vi "Teleop.vi"(10 "Match Info":T1={"Autonomous Elapsed Seconds"=0.0, "TeleOp Elapsed Seconds"=0.0, "Disabled Elapsed Seconds"=0.0, "Visited Autonomous"=FALSE, "Visited TeleOp"=FALSE, "Visited Disabled"=FALSE, "Autonomous Settings"={"Autonomous Style"=enum."Independent", "VI Refnum"=refnum}}, 11 "Call Context":T2) -> ()   [LabVIEW 2020]
doc: "This VI is called for each TeleOp packet received from the DS where the robot is not disabled. It is often used to read from the joysticks and update I/O or to update setpoints for timed control loops. It should complete and return within 20 milliseconds or it may miss DS packets."
uses:
  <vilib>/Rock Robotics/WPI/DriverStation/WPI_DriverStationDerivedRobotMode.ctl
  <vilib>/Rock Robotics/WPI/DriverStation/WPI_DriverStationMatch Info.ctl
  <vilib>/Rock Robotics/WPI/ThirdParty/Phoenix-LabVIEW/Motor Controller/Controls/CTRE_Phoenix_MotorControl_ControlMode.ctl
  <vilib>/Rock Robotics/WPI/Solenoid/WPI_SolenoidValue.ctl
  <vilib>/Rock Robotics/WPI/Utilities/WPI_GetSetVariantRefNum.vi
  <vilib>/Rock Robotics/Network Tables/NT Write Boolean Array.vi
  <vilib>/Rock Robotics/Network Tables/NT Write Numeric Array.vi
  <vilib>/Rock Robotics/Network Tables/NT Read Boolean.vi
  <vilib>/Rock Robotics/WPI/Solenoid/WPI_SolenoidSetEnum.vi
  <vilib>/Rock Robotics/WPI/ThirdParty/Phoenix-LabVIEW/Motor Controller/Get/CTRE_Phoenix_MotorController_IntegratedSensorData_TalonFX.vi
  <vilib>/Rock Robotics/WPI/ThirdParty/Phoenix-LabVIEW/Motor Controller/Get/CTRE_Phoenix_MotorController_GetLimitSwitchStates.vi
  <vilib>/Rock Robotics/WPI/ThirdParty/Phoenix-LabVIEW/Motor Controller/Sensor/CTRE_Phoenix_MotorControl_SetIntegratedSensorPosition_TalonFX.vi
  <vilib>/Rock Robotics/Network Tables/NT Write Number.vi
  Lime.vi
  <vilib>/Rock Robotics/WPI/RobotDrive/WPI_RobotDriveMecanumDrive_Cartesian.vi
panel:
  in  "Numeric":dbl=-0.7 format="%#_13g"
  in  "Auger Speed":dbl=-0.8
  out "Present Text":string
  in  "Total Time":dbl=0.9 format="%#_13g"
  in  "Time Low":dbl=0.6 format="%#_13g"
  in  "Slowmode Speed":dbl=0.33
  out "Compressor Running":bool
  out "Enabled":bool
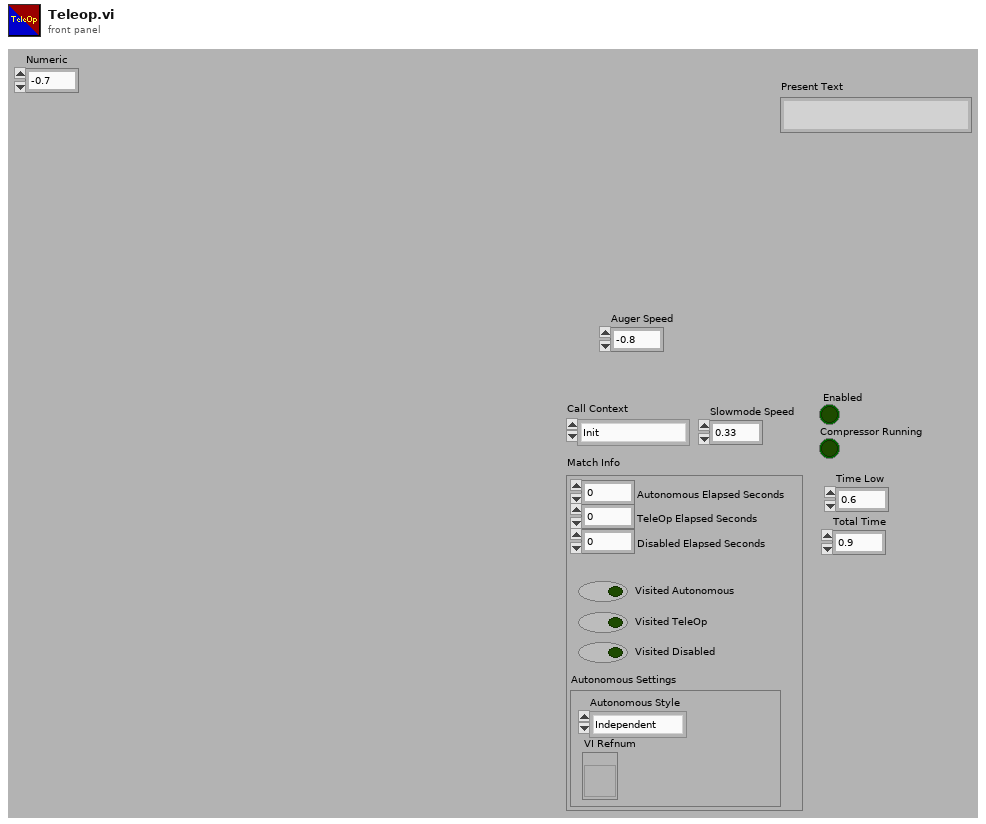
[diagram p1: front panel]
types:
  T1 = typedef "WPI_DriverStationMatch Info.ctl" = cluster{"Autonomous Elapsed Seconds":dbl, "TeleOp Elapsed Seconds":dbl, "Disabled Elapsed Seconds":dbl, "Visited Autonomous":bool, "Visited TeleOp":bool, "Visited Disabled":bool, "Autonomous Settings":cluster{"Autonomous Style":enum16{"Iterative", "Independent"}, "VI Refnum":refnum<vi>}}
  T2 = typedef "WPI_DriverStationDerivedRobotMode.ctl" = enum16{"Init", "Execute", "Stop"}
  T3 = typedef "WPI_SolenoidValue.ctl" = enum16{"Off", "On", "Forward", "Reverse"}
  T4 = typedef "CTRE_Phoenix_MotorControl_ControlMode.ctl" = u16
  T5 = typedef "WPI_JoystickDevRef.ctl" = cluster{"Device":T6}
  T6 = typedef "WPI_JoystickDeviceEnum.ctl" = enum16{"USB 0", "USB 1", "USB 2", "USB 3", "USB 4", "USB 5"}
  T7 = typedef "WPI_CompressorDevRef.ctl" = cluster{"DevStatus":errorcluster, "Pneumatics Control Module":u8}
  T8 = typedef "WPI_RobotDriveDevRef.ctl" = cluster{"DevStatus":errorcluster, "Motors[]":T9[], "Square Inputs":bool, "Max Output":dbl}
  T9 = typedef "WPI_MotorControlDeviceRef.ctl" = cluster{"DeviceStatus":errorcluster, "Type":T10, "PWM":cluster{"PWM Channel":T11, "DeadBand":T12}, "CAN":cluster{"Device Number":u8, "SetOutput VI Ref":variant, "GetOutput VI Ref":variant, "Enable VI Ref":variant, "Disable VI Ref":variant, "Data":variant}, "Invert":bool, "DIO PWM":cluster{"PWM \"Enable\" Channel":T11, "DIOChannel":T13, "PWM Rate":dbl}}
  T10 = typedef "WPI_MotorControlType.ctl" = enum16{"PWM", "CAN", "DIO PWM"}
  T11 = typedef "FPGA_DIOPWMChannel.ctl" = enum8{"PWM 0", "PWM 1", "PWM 2", "PWM 3", "PWM 4", "PWM 5", "PWM 6", "PWM 7", "PWM 8", "PWM 9", "PWM MXP 0", "PWM MXP 1", "PWM MXP 2", "PWM MXP 3", "PWM MXP 4", "PWM MXP 5", "PWM MXP 6", "PWM MXP 7", "PWM MXP 8", "PWM MXP 9", "Invalid"}
  T12 = typedef "WPI_PWMDeadband.ctl" = cluster{"Name":string, "maxPositivePwm":i32, "minPositivePwm":i32, "centerPwm":i32, "maxNegativePwm":i32, "minNegativePwm":i32, "angularRange":u16}
  T13 = typedef "FPGA_DIOChannel.ctl" = enum8{"DIO 0", "DIO 1", "DIO 2", "DIO 3", "DIO 4", "DIO 5", "DIO 6", "DIO 7", "DIO 8", "DIO 9", "DIO MXP 0", "DIO MXP 1", "DIO MXP 2", "DIO MXP 3", "DIO MXP 4", "DIO MXP 5", "DIO MXP 6", "DIO MXP 7", "DIO MXP 8", "DIO MXP 9", "DIO MXP 10", "DIO MXP 11", "DIO MXP 12", "DIO MXP 13", "DIO MXP 14", "DIO MXP 15", "SPI Port CS1", "SPI Port CS2", "SPI Port CS3", "SPI Port MISO", "SPI Port MOSI", "Invalid"}
  T14 = typedef "WPI_DigitalInputDevRef.ctl" = cluster{"DevStatus":errorcluster, "DIO Channel":T13}
  T15 = typedef "WPI_SolenoidDevRef.ctl" = cluster{"DevStatus":errorcluster, "Pneumatics Control Module":u8, "Forward Solenoid Channel":T16, "Reverse Solenoid Channel":T16}
  T16 = typedef "WPI_SolenoidChannel.ctl" = enum8{"Solenoid 0", "Solenoid 1", "Solenoid 2", "Solenoid 3", "Solenoid 4", "Solenoid 5", "Solenoid 6", "Solenoid 7", "Solenoid 8", "Solenoid 9", "Solenoid 10", "Solenoid 11", "Solenoid 12", "Solenoid 13", "Solenoid 14", "Solenoid 15", "Invalid"}
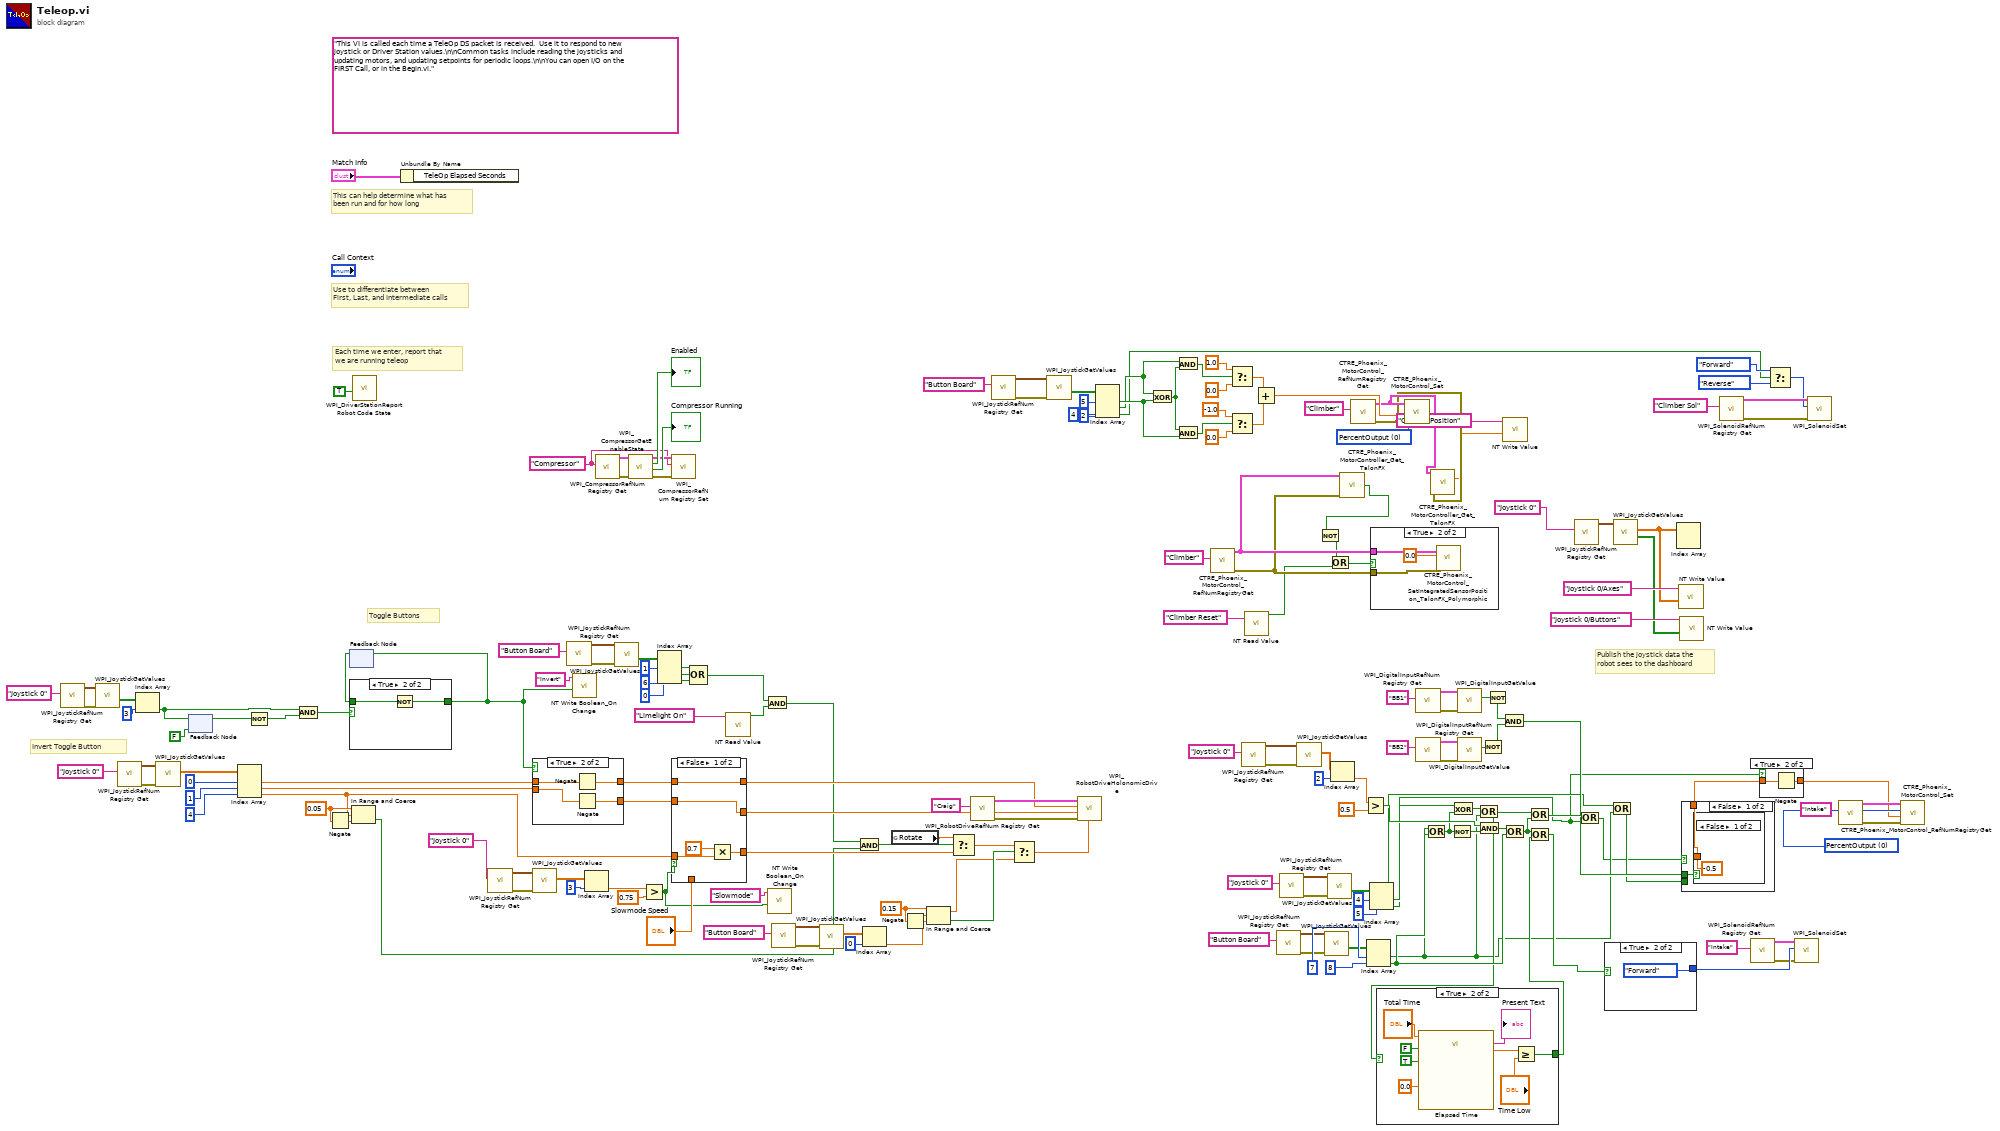
[diagram p0: block diagram]
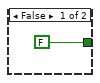
[diagram p4: hidden frame]
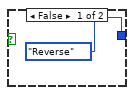
[diagram p5: hidden frame]
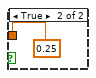
[diagram p6: hidden frame]
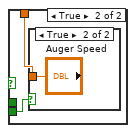
[diagram p7: hidden frame]
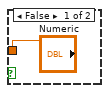
[diagram p8: hidden frame]
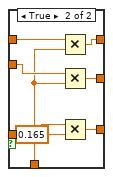
[diagram p9: hidden frame]
diagram:
  w41 = T4 0 items=["PercentOutput"=0, "Position"=1, "Velocity"=2, "Current"=3, "Follower"=5, "MotionProfile"=6, "MotionMagic"=7, "MotionProfileArc"=10, "Disabled"=15] ("Control Mode")
  w45 = 0.15 ("upper limit")
  w56 = 0.05 ("upper limit")
  w91 = T4 0 items=["PercentOutput"=0, "Position"=1, "Velocity"=2, "Current"=3, "Follower"=5, "MotionProfile"=6, "MotionMagic"=7, "MotionProfileArc"=10, "Disabled"=15] ("Control Mode")
  w169 = "Compressor" ("refnum name")
  (unwired) "This VI is called each time a TeleOp DS packet is received.  Use it to respond to new joystick or Driver Station values.\n\nCommon tasks include reading the joysticks and updating motors, and updating setpoints for periodic loops.\n\nYou can open I/O on the FIRST Call, or in the Begin.vi."
  # "Invert Toggle Button"
  # "Toggle Buttons"
  # "Publish the joystick data the\nrobot sees to the dashboard"
  # "Each time we enter, report that\nwe are running teleop"
  # "Use to differentiate between\nFirst, Last, and Intermediate calls"
  # "This can help determine what has\nbeen run and for how long"
  n1 = call <vilib>:"WPI_JoystickRefNum Registry Get.vi"("refnum name"="Joystick 0") -> ("error out"=w158:errorcluster, "JoystickDevRef"=w147:T5)  [unwired: 9 in]
  n2 = call <vilib>:"WPI_JoystickGetValues.vi"("error in (no error)"=w158, "JoystickDevRef"=w147) -> ("Buttons"=w155:bool[])  [unwired: 5 in, 4 out]
  n3 = call <vilib>:"WPI_JoystickRefNum Registry Get.vi"("refnum name"="Joystick 0") -> ("error out"=w165:errorcluster, "JoystickDevRef"=w166:T5)  [unwired: 9 in]
  n4 = Index Array(array=w155, index=3) -> (element=w149:bool)
  n5 = call <vilib>:"WPI_JoystickGetValues.vi"("error in (no error)"=w165, "JoystickDevRef"=w166) -> ("Axes"=w162:dbl[])  [unwired: 5 in, 4 out]
  n6 = feedback #1(FALSE) -> (w151:bool)
  n7 = feedback-in #1(w149) -> ()
  n8 = Index Array(array=w162, index #1=0 ("index"), index #2=1 ("index"), index #3=4 ("index")) -> (element #1=w148:dbl, element #2=w135:dbl, element #3=w53:dbl)
  n9 = Not(x=w151) -> (.not. x?=w152:bool)
  n10 = And(x=w149, y=w152) -> (x .and. y?=w153:bool)
  n11 = Negate(x=w56) -> (-x=w57:dbl)
  n12 = feedback #2() -> (w154:bool)  [unwired: 1 in]
  n13 = case shown="True" w153 {
    tunnel: w154 -> [w184 w186]
    tunnel: [w184 w185] -> w134
    frame False {
    }
    frame True {
      n14 = Not(x=w186) -> (.not. x?=w185:bool)
    }
  }
  n15 = feedback-in #2(w134) -> ()
  n16 = In Range and Coerce(upper limit=w56, x=w53, lower limit=w57) -> (In Range?=w54:bool)  [unwired: 1 out]
  n17 = call <vilib>:"WPI_DriverStationReport Robot Code State.vi"("TeleOp"=TRUE ("Autonomous")) -> ()  [unwired: 10 in, 1 out]
  n18 = Unbundle By Name("Match Info") -> ()  [unwired: 1 out]
  n19 = call <vilib>:"WPI_JoystickRefNum Registry Get.vi"("refnum name"="Joystick 0") -> ("error out"=w141:errorcluster, "JoystickDevRef"=w144:T5)  [unwired: 9 in]
  n20 = case shown="True" w134 {
    tunnel: [w188 w189] -> w146
    tunnel: w148 -> [w188 w190]
    tunnel: [w187 w191] -> w145
    tunnel: w135 -> [w187 w192]
    frame False {
    }
    frame True {
      n21 = Negate(x=w190) -> (-x=w189:dbl)
      n22 = Negate(x=w192) -> (-x=w191:dbl)
    }
  }
  n23 = call <vilib>:"WPI_JoystickGetValues.vi"("error in (no error)"=w141, "JoystickDevRef"=w144) -> ("Axes"=w140:dbl[])  [unwired: 5 in, 4 out]
  n24 = call <vilib>:"WPI_JoystickRefNum Registry Get.vi"("refnum name"="Button Board") -> ("error out"=w129:errorcluster, "JoystickDevRef"=w127:T5)  [unwired: 9 in]
  n25 = call "NT Write Boolean_On Change.vi"("Boolean"=w134, "Name"="Invert") -> ()  [unwired: 9 in, 1 out]
  n26 = Index Array(array=w140, index=3) -> (element=w139:dbl)
  n27 = call <vilib>:"WPI_CompressorRefNum Registry Get.vi"("refnum name"=w169) -> ("error out"=w173:errorcluster, "CompressorDevRef"=w172:T7)  [unwired: 9 in]
  n28 = call <vilib>:"WPI_JoystickGetValues.vi"("error in (no error)"=w129, "JoystickDevRef"=w127) -> ("Buttons"=w128:bool[])  [unwired: 5 in, 4 out]
  n29 = call <vilib>:"WPI_CompressorGetEnableState.vi"("error in (no error)"=w173, "CompressorDevRef"=w172) -> ("error out"=w170:errorcluster, "Compressor Running"=→"Compressor Running":bool, "Enabled"=→"Enabled":bool, "CompressorDevRef"=w171:T7)  [unwired: 3 in, 3 out]
  n30 = Greater?(x=w139, y=0.75) -> (0:w131:bool)
  n31 = Index Array(array=w128, index #1=1 ("index"), index #2=6 ("index"), index #3=0 ("index")) -> (element #1=w120:bool, element #2=w122:bool, element #3=w121:bool)
  n32 = call <vilib>:"WPI_CompressorRefNum Registry Set.vi"("error in (no error)"=w170, "refnum name"=w169, "CompressorDevRef"=w171) -> ()  [unwired: 7 in, 2 out]
  n33 = case shown="False" w131 {
    tunnel: w53 -> [w197 w205]
    tunnel: [w194 w204] -> w59
    tunnel: w146 -> [w196 w203]
    tunnel: [w196 w202] -> w137
    tunnel: w145 -> [w195 w201]
    tunnel: [w195 w200] -> w123
    tunnel: "Slowmode Speed" -> [_ w199]
    frame False {
      n34 = Multiply(x=0.7, y=w197) -> (x*y=w194:dbl)
    }
    frame True {
      n35 = Multiply(x=w203, y=w199) -> (x*y=w202:dbl)
      n36 = Multiply(x=w201, y=w199) -> (x*y=w200:dbl)
      n37 = Multiply(x=w205, y=0.165) -> (x*y=w204:dbl)
    }
  }
  n38 = Compound Arithmetic op=OR(w120, w122, w121) -> (w117:bool)
  n39 = call-poly <vilib>:"NT Read Value.vi"("Name"="Limelight On") -> ("Boolean"=w119:bool)  [unwired: 9 in, 1 out]
  n40 = And(x=w117, y=w119) -> (x .and. y?=w61:bool)
  n41 = call "NT Write Boolean_On Change.vi"("Boolean"=w131, "Name"="Slowmode") -> ()  [unwired: 9 in, 1 out]
  n42 = call <vilib>:"WPI_JoystickRefNum Registry Get.vi"("refnum name"="Button Board") -> ("error out"=w50:errorcluster, "JoystickDevRef"=w51:T5)  [unwired: 9 in]
  n43 = call <vilib>:"WPI_JoystickGetValues.vi"("error in (no error)"=w50, "JoystickDevRef"=w51) -> ("Axes"=w48:dbl[])  [unwired: 5 in, 4 out]
  n44 = And(x=w61, y=w54) -> (x .and. y?=w55:bool)
  n45 = Index Array(array=w48, index=0) -> (element=w44:dbl)
  n46 = global read "Lime.vi" "Rotate"() -> (w60:dbl)
  n47 = Negate(x=w45) -> (-x=w47:dbl)
  n48 = In Range and Coerce(upper limit=w45, x=w44, lower limit=w47) -> (coerced(x)=w42:dbl, In Range?=w46:bool)
  n49 = Select(t=w60, s=w55, f=w59) -> (s? t:f=w58:dbl)
  n50 = call <vilib>:"WPI_RobotDriveRefNum Registry Get.vi"("refnum name"="Craig") -> ("error out"=w167:errorcluster, "RobotDriveDevRef"=w168:T8)  [unwired: 9 in]
  n51 = call <vilib>:"WPI_JoystickRefNum Registry Get.vi"("refnum name"="Button Board") -> ("error out"=w38:errorcluster, "JoystickDevRef"=w39:T5)  [unwired: 9 in]
  n52 = Select(t=w58, s=w46, f=w42) -> (s? t:f=w43:dbl)
  n53 = call <vilib>:"WPI_JoystickGetValues.vi"("error in (no error)"=w38, "JoystickDevRef"=w39) -> ("Buttons"=w36:bool[])  [unwired: 5 in, 4 out]
  n54 = call-poly <vilib>:"WPI_RobotDriveHolonomicDrive.vi"("Rotation"=w43, "error in (no error)"=w167, "Y"=w123, "X"=w137, "RobotDriveDevRef"=w168) -> ()  [unwired: 4 in, 3 out]
  n55 = Index Array(array=w36, index #1=5 ("index"), index #2=2 ("index"), index #3=4 ("index")) -> (element #1=w24:bool, element #2=w23:bool, element #3=w2:bool)
  n56 = Exclusive Or(1:w24, 2:w23) -> (0:w27:bool)
  n57 = And(x=w23, y=w27) -> (x .and. y?=w29:bool)
  n58 = And(x=w27, y=w24) -> (x .and. y?=w28:bool)
  n59 = call <vilib>:"CTRE_Phoenix_MotorControl_RefNumRegistryGet.vi"("refnum name"="Climber") -> ("error out"=w19:errorcluster, "PhoenixMotorControlDevRef"=w20:T9)  [unwired: 9 in]
  n60 = Select(t=1.0, s=w29, f=0.0) -> (s? t:f=w25:dbl)
  n61 = Select(t=-1.0, s=w28, f=0.0) -> (s? t:f=w26:dbl)
  n62 = call <vilib>:"WPI_JoystickRefNum Registry Get.vi"("refnum name"="Joystick 0") -> ("error out"=w96:errorcluster, "JoystickDevRef"=w95:T5)  [unwired: 9 in]
  n63 = call-poly <vilib>:"NT Read Value.vi"("Name"="Climber Reset") -> ("Boolean"=w15:bool)  [unwired: 9 in, 1 out]
  n64 = Add(x=w25, y=w26) -> (x+y=w22:dbl)
  n65 = call <vilib>:"WPI_JoystickRefNum Registry Get.vi"("refnum name"="Button Board") -> ("error out"=w79:errorcluster, "JoystickDevRef"=w77:T5)  [unwired: 9 in]
  n66 = call <vilib>:"WPI_JoystickRefNum Registry Get.vi"("refnum name"="Joystick 0") -> ("error out"=w102:errorcluster, "JoystickDevRef"=w104:T5)  [unwired: 9 in]
  n67 = call <vilib>:"WPI_JoystickGetValues.vi"("error in (no error)"=w96, "JoystickDevRef"=w95) -> ("Axes"=w97:dbl[])  [unwired: 5 in, 4 out]
  n68 = call <vilib>:"WPI_JoystickGetValues.vi"("error in (no error)"=w79, "JoystickDevRef"=w77) -> ("Buttons"=w78:bool[])  [unwired: 5 in, 4 out]
  n69 = call <vilib>:"WPI_JoystickGetValues.vi"("error in (no error)"=w102, "JoystickDevRef"=w104) -> ("Buttons"=w103:bool[])  [unwired: 5 in, 4 out]
  n70 = Index Array(array=w97, index=2) -> (element=w98:dbl)
  n71 = call-poly <vilib>:"CTRE_Phoenix_MotorController_Get_TalonFX.vi"("PhoenixMotorControlDevRef"=w20, "error in"=w19) -> ("Reverse Limit Closed?"=w18:bool)  [unwired: 10 in, 3 out]
  n72 = Not(x=w18) -> (.not. x?=w17:bool)
  n73 = Or(x=w17, y=w15) -> (x .or. y?=w16:bool)
  n74 = call <vilib>:"CTRE_Phoenix_MotorControl_RefNumRegistryGet.vi"("refnum name"="Climber") -> ("error out"=w12:errorcluster, "PhoenixMotorControlDevRef"=w13:T9)  [unwired: 9 in]
  n75 = Greater?(x=w98, y=0.5) -> (0:w72:bool)
  n76 = Index Array(array=w78, index #1=7 ("index"), index #2=8 ("index")) -> (element #1=w66:bool, element #2=w73:bool)
  n77 = Index Array(array=w103, index #1=4 ("index"), index #2=5 ("index")) -> (element #1=w67:bool, element #2=w1:bool)
  n78 = case shown="True" w16 {
    tunnel: w20 -> [_ w208]
    tunnel: w19 -> [_ w207]
    frame False {
    }
    frame True {
      n79 = call-poly <vilib>:"CTRE_Phoenix_MotorControl_SetIntegratedSensorPosition_TalonFX_Polymorphic.vi"("error in (no error)"=w207, "New Position"=0.0, "PhoenixMotorControlDevRef"=w208) -> ()  [unwired: 7 in, 2 out]
    }
  }
  n80 = call <vilib>:"CTRE_Phoenix_MotorControl_Set.vi"("error in (no error)"=w12, "Output"=w22, "Control Mode"=w41, "PhoenixMotorControlDevRef"=w13) -> ()  [unwired: 6 in, 2 out]
  n81 = call <vilib>:"WPI_DigitalInputRefNum Registry Get.vi"("refnum name"="BB1") -> ("error out"=w116:errorcluster, "DigitalInputDevRef"=w115:T14)  [unwired: 9 in]
  n82 = call <vilib>:"WPI_DigitalInputRefNum Registry Get.vi"("refnum name"="BB2") -> ("error out"=w113:errorcluster, "DigitalInputDevRef"=w112:T14)  [unwired: 9 in]
  n83 = Or(x=w66, y=w73) -> (x .or. y?=w69:bool)
  n84 = call-poly <vilib>:"CTRE_Phoenix_MotorController_Get_TalonFX.vi"("PhoenixMotorControlDevRef"=w13, "error in"=w12) -> ("Position"=w10:dbl)  [unwired: 9 in, 4 out]
  n85 = Not(x=w69) -> (.not. x?=w70:bool)
  n86 = Exclusive Or(1:w69, 2:w67) -> (0:w75:bool)
  n87 = call <vilib>:"WPI_DigitalInputGetValue.vi"("error in (no error)"=w116, "DigitalInputDevRef"=w115) -> ("Value"=w110:bool)  [unwired: 7 in, 2 out]
  n88 = call <vilib>:"WPI_DigitalInputGetValue.vi"("error in (no error)"=w113, "DigitalInputDevRef"=w112) -> ("Value"=w109:bool)  [unwired: 7 in, 2 out]
  n89 = Or(x=w75, y=w66) -> (x .or. y?=w68:bool)
  n90 = case shown="True" w68 {
    tunnel: [FALSE w210] -> w83
    frame False {
    }
    frame True {
      n91 = call "Elapsed Time"("Time Target (s)"="Total Time", "Reset"=FALSE, "Auto Reset"=TRUE, "Set Start Time (s)"=0.0) -> ("Present Text"=→"Present Text":string, "Elapsed Time (s)"=w212:dbl)  [unwired: 8 in, 6 out]
      n92 = Greater Or Equal?(x=w212, y="Time Low") -> (x >= y?=w210:bool)
    }
  }
  n93 = And(x=w72, y=w70) -> (x .and. y?=w71:bool)
  n94 = Not(x=w109) -> (.not. x?=w107:bool)
  n95 = Not(x=w110) -> (.not. x?=w108:bool)
  n96 = And(x=w108, y=w107) -> (x .and. y?=w85:bool)
  n97 = call-poly <vilib>:"NT Write Value.vi"("Numeric"=w10, "Name"="Climber Position") -> ()  [unwired: 9 in, 1 out]
  n98 = Or(x=w71, y=w73) -> (x .or. y?=w74:bool)
  n99 = Or(x=w68, y=w74) -> (x .or. y?=w106:bool)
  n100 = Or(x=w74, y=w83) -> (x .or. y?=w84:bool)
  n101 = call <vilib>:"WPI_JoystickRefNum Registry Get.vi"("refnum name"="Joystick 0") -> ("JoystickDevRef"=w181:T5)  [unwired: 1 in, 9 out]
  n102 = Or(x=w106, y=w1) -> (x .or. y?=w62:bool)
  n103 = case shown="True" w84 {
    tunnel: [WPI_SolenoidValue."Reverse" ("Value") WPI_SolenoidValue."Forward" ("Value")] -> w105
    frame False {
    }
    frame True {
    }
  }
  n104 = Or(x=w67, y=w66) -> (x .or. y?=w65:bool)
  n105 = call <vilib>:"WPI_JoystickGetValues.vi"("JoystickDevRef"=w181) -> ("Buttons"=w176:bool[], "Axes"=w177:dbl[])  [unwired: 6 in, 3 out]
  n106 = Index Array(array=w177) -> ()  [unwired: 2 in, 2 out]
  n107 = call-poly <vilib>:"NT Write Value.vi"("Numeric Array"=w177, "Name"="Joystick 0/Axes") -> ()  [unwired: 9 in, 1 out]
  n108 = call-poly <vilib>:"NT Write Value.vi"("Boolean Array"=w176, "Name"="Joystick 0/Buttons") -> ()  [unwired: 9 in, 1 out]
  n109 = case shown="False" w62 {
    tunnel: [w221 w225] -> w101
    tunnel: w85 -> [w220 _]
    tunnel: w65 -> [_ w224]
    frame False {
      n110 = case shown="False" w220 {
        tunnel: [-0.5 0.25] -> w221
        frame False {
        }
        frame True {
        }
      }
    }
    frame True {
      n111 = case shown="True" w224 {
        tunnel: ["Numeric" "Auger Speed"] -> w225
        frame False {
        }
        frame True {
        }
      }
    }
  }
  n112 = call <vilib>:"WPI_SolenoidRefNum Registry Get.vi"("refnum name"="Climber Sol") -> ("error out"=w7:errorcluster, "SolenoidDevRef"=w9:T15)  [unwired: 9 in]
  n113 = call <vilib>:"WPI_SolenoidRefNum Registry Get.vi"("refnum name"="Intake") -> ("error out"=w94:errorcluster, "SolenoidDevRef"=w93:T15)  [unwired: 9 in]
  n114 = case shown="True" w1 {
    tunnel: w101 -> [w228 w230]
    tunnel: [w228 w229] -> w63
    frame False {
    }
    frame True {
      n115 = Negate(x=w230) -> (-x=w229:dbl)
    }
  }
  n116 = Select(t=WPI_SolenoidValue."Forward" ("Value"), s=w2, f=WPI_SolenoidValue."Reverse" ("Value")) -> (s? t:f=w4:T3)
  n117 = call-poly <vilib>:"WPI_SolenoidSet.vi"("error in (no error)"=w94, "Value"=w105, "SolenoidDevRef"=w93) -> ()  [unwired: 7 in, 2 out]
  n118 = call-poly <vilib>:"WPI_SolenoidSet.vi"("error in (no error)"=w7, "Value"=w4, "SolenoidDevRef"=w9) -> ()  [unwired: 7 in, 2 out]
  n119 = call <vilib>:"CTRE_Phoenix_MotorControl_RefNumRegistryGet.vi"("refnum name"="Intake") -> ("error out"=w100:errorcluster, "PhoenixMotorControlDevRef"=w99:T9)  [unwired: 9 in]
  n120 = call <vilib>:"CTRE_Phoenix_MotorControl_Set.vi"("error in (no error)"=w100, "Output"=w63, "Control Mode"=w91, "PhoenixMotorControlDevRef"=w99) -> ()  [unwired: 6 in, 2 out]
